vi "x-axis.vi"(8 "error in (no error)":errorcluster, 11 "Pulse Gen Basic Scan in":refnum<class "Pulse Gen Basic Scan.lvclass">) -> (0 "error out":errorcluster, 1 "Label":string, 2 "Unit":string, 3 "Pulse Gen Basic Scan out":refnum<class "Pulse Gen Basic Scan.lvclass">)   [LabVIEW 2023, in "Pulse Gen Basic Scan.lvclass"]
uses:
  Pulse Gen Basic Scan.lvclass
  Scanner/Scanner.lvclass
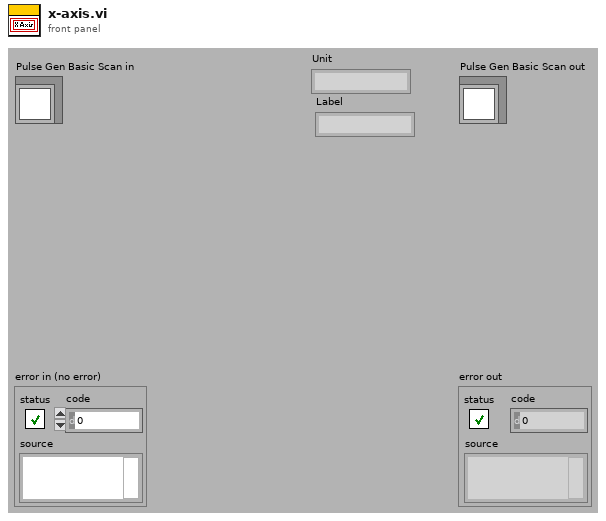
[diagram p1: front panel]
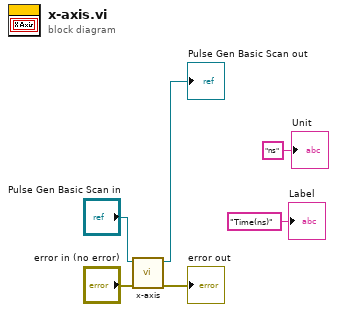
[diagram p0: block diagram]
diagram:
  n1 = call-parent "x-axis.vi"("error in (no error)"="error in (no error)", "Scanner in"="Pulse Gen Basic Scan in") -> ("error out"=→"error out":errorcluster, "Scanner out"=→"Pulse Gen Basic Scan out":refnum<class "Pulse Gen Basic Scan.lvclass">)  [unwired: 6 in, 2 out]
  "Label" <- "Time(ns)" ("Label")
  "Unit" <- "ns" ("Unit")
